vi "Stop Static.vi"(8 "error in (no error)":errorcluster, 11 "Actor in":refnum<class "Actor.lvclass">) -> (0 "error out":errorcluster, 3 "Actor out":refnum<class "Actor.lvclass">)   [LabVIEW 2020, in "Artifex.lvlib" / "Actor.lvclass"]
uses:
  Actor.lvclass
  Actor Proxy/Actor API.lvclass
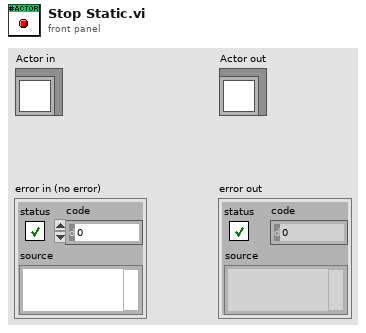
[diagram p1: front panel]
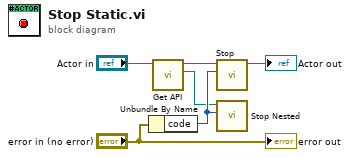
[diagram p0: block diagram]
diagram:
  n1 = Unbundle By Name("error in (no error)") -> ("code"=w6:i32)
  n2 = call-dynamic "Get API.vi"("Actor in"="Actor in") -> ("Actor API"=w3:refnum<class "Actor API.lvclass">, "Actor out"=w4:refnum<class "Actor.lvclass">)  [unwired: 8 in, 1 out]
  n3 = call-dynamic "Stop.vi"("Code"=w6, "Actor in"=w4) -> ("Actor out"=→"Actor out":refnum<class "Actor.lvclass">)  [unwired: 9 in]
  n4 = call "Stop Nested.vi"("Final Code"=w6, "Actor API in"=w3) -> ()  [unwired: 9 in, 1 out]
  "error out" <- "error in (no error)"
